vi "picoscope_910nm hitung distance_kompensasi gain.vi"() -> ()   [LabVIEW 2016]
doc: "This example demonstrates how to continuously re-generate analog output data from a buffer in your computer's memory.\n\nRefer to your device documentation for pinouts and hardware capabilities."
uses:
  <vilib>/Analysis/coordinate.llb/Angle Units.ctl
  <vilib>/Analysis/coordinate.llb/Angle Range (Degree).ctl
  <vilib>/Analysis/baseanly.llb/Mean (DBL).vi
  <vilib>/Analysis/coordinate.llb/Wrap Angle (scalar).vi
  <vilib>/measure/mascope.llb/Pulse Measurements 1 chan.vi
  <vilib>/measure/matone.llb/Extract Single Tone Information 1 Chan.vi
  <vilib>/measure/NI_MAPro.lvlib
  <vilib>/Analysis/NI_AAL_Angle.lvlib
  <vilib>/Analysis/NI_AALBase.lvlib
panel:
  in  "Channel C":T1={"Enabled"=TRUE, "DC Coupled"=FALSE, "Range"=6} {"Range" items=["10 mV", "20 mV", "50 mV", "100 mV", "200 mV", "500 mV", "1 V", "2 V", "5 V", "10 V", "20 V", "50 V ", "100 V"]}
  in  "Reset saving":bool caption="Reset"
  in  "Acquisition Settings":T2={"preTriggerSamples"=0, "postTriggerSamples"=1000, "timebase"=2, "Aggregate Data"=FALSE, "Down Sample Ratio"=1, "Four Channel Device"=TRUE, "Oversample"=1} {"Down Sample Ratio" min=1 step=1}
  in  "Channel A":T1={"Enabled"=TRUE, "DC Coupled"=FALSE, "Range"=6} {"Range" items=["10 mV", "20 mV", "50 mV", "100 mV", "200 mV", "500 mV", "1 V", "2 V", "5 V", "10 V", "20 V", "50 V ", "100 V"]}
  in  "Phase Measurement":enum32{"Square", "Sinusoidal"}(tab)
  out "Time Shift 3":dbl
  out "Pulse center 3":dbl
  out "Pulse Center 2":dbl
  out "Phase Shift 2":dbl
  out "Ref frequency":dbl format="%.2p"
  out "Signal frequency":dbl format="%.2p"
  out "Amp A":dbl format="%.2g"
  out "Amp C":dbl format="%_3g"
  out "Phase total":dbl format="%#_4g"
  out "Phase 2 M":dbl format="%0.2f"
  out "Phase 10 M":dbl format="%0.2f"
  out "Validation":string="not range"
  out "Distance (m)":dbl format="%#.3g"
  in  "Enable Av_Gain":bool
  in  "Save":bool caption="Enable"
  out "Waveform Graph":dbl[][](graph) caption="Output Waveform"
  in  "Stop":bool
  out "phase sbl":dbl
  out "Phase Shift (deg)":dbl
  out "phase 2 (2M)":dbl
  out "phase 1 (10M)":dbl
  out "mean phase 10 M":dbl format="%0.2f"
  out "Array 2":dbl[](array[numeric])
  out "number 2":u32
  out "mean phase 2 M":dbl format="%0.2f"
  out "Array":dbl[](array[numeric])
  out "Phase signal":dbl
  out "number":u32
  out "appended array":bool[](array[boolean])
  out "DC RMS":dbl format="%#_3g"
  out "Data out":dbl[](array[numeric])
  out "Phase Signal ref":dbl
  in  "Channel D Settings":T1={"Enabled"=FALSE, "DC Coupled"=TRUE, "Range"=6} {"Range" items=["10 mV", "20 mV", "50 mV", "100 mV", "200 mV", "500 mV", "1 V", "2 V", "5 V", "10 V", "20 V", "50 V ", "100 V"]}
  in  "Channel B Settings":T1={"Enabled"=FALSE, "DC Coupled"=FALSE, "Range"=6} {"Range" items=["10 mV", "20 mV", "50 mV", "100 mV", "200 mV", "500 mV", "1 V", "2 V", "5 V", "10 V", "20 V", "50 V ", "100 V"]}
  # "median"
  # "Channel Settings"
  # "Trigger Settings"
  # "1   2   4   8   16  32 64 128  256 512 1024  2028"
  # "OPI i-ToF LiDAR\nResearch Center for Photonics - BRIN"
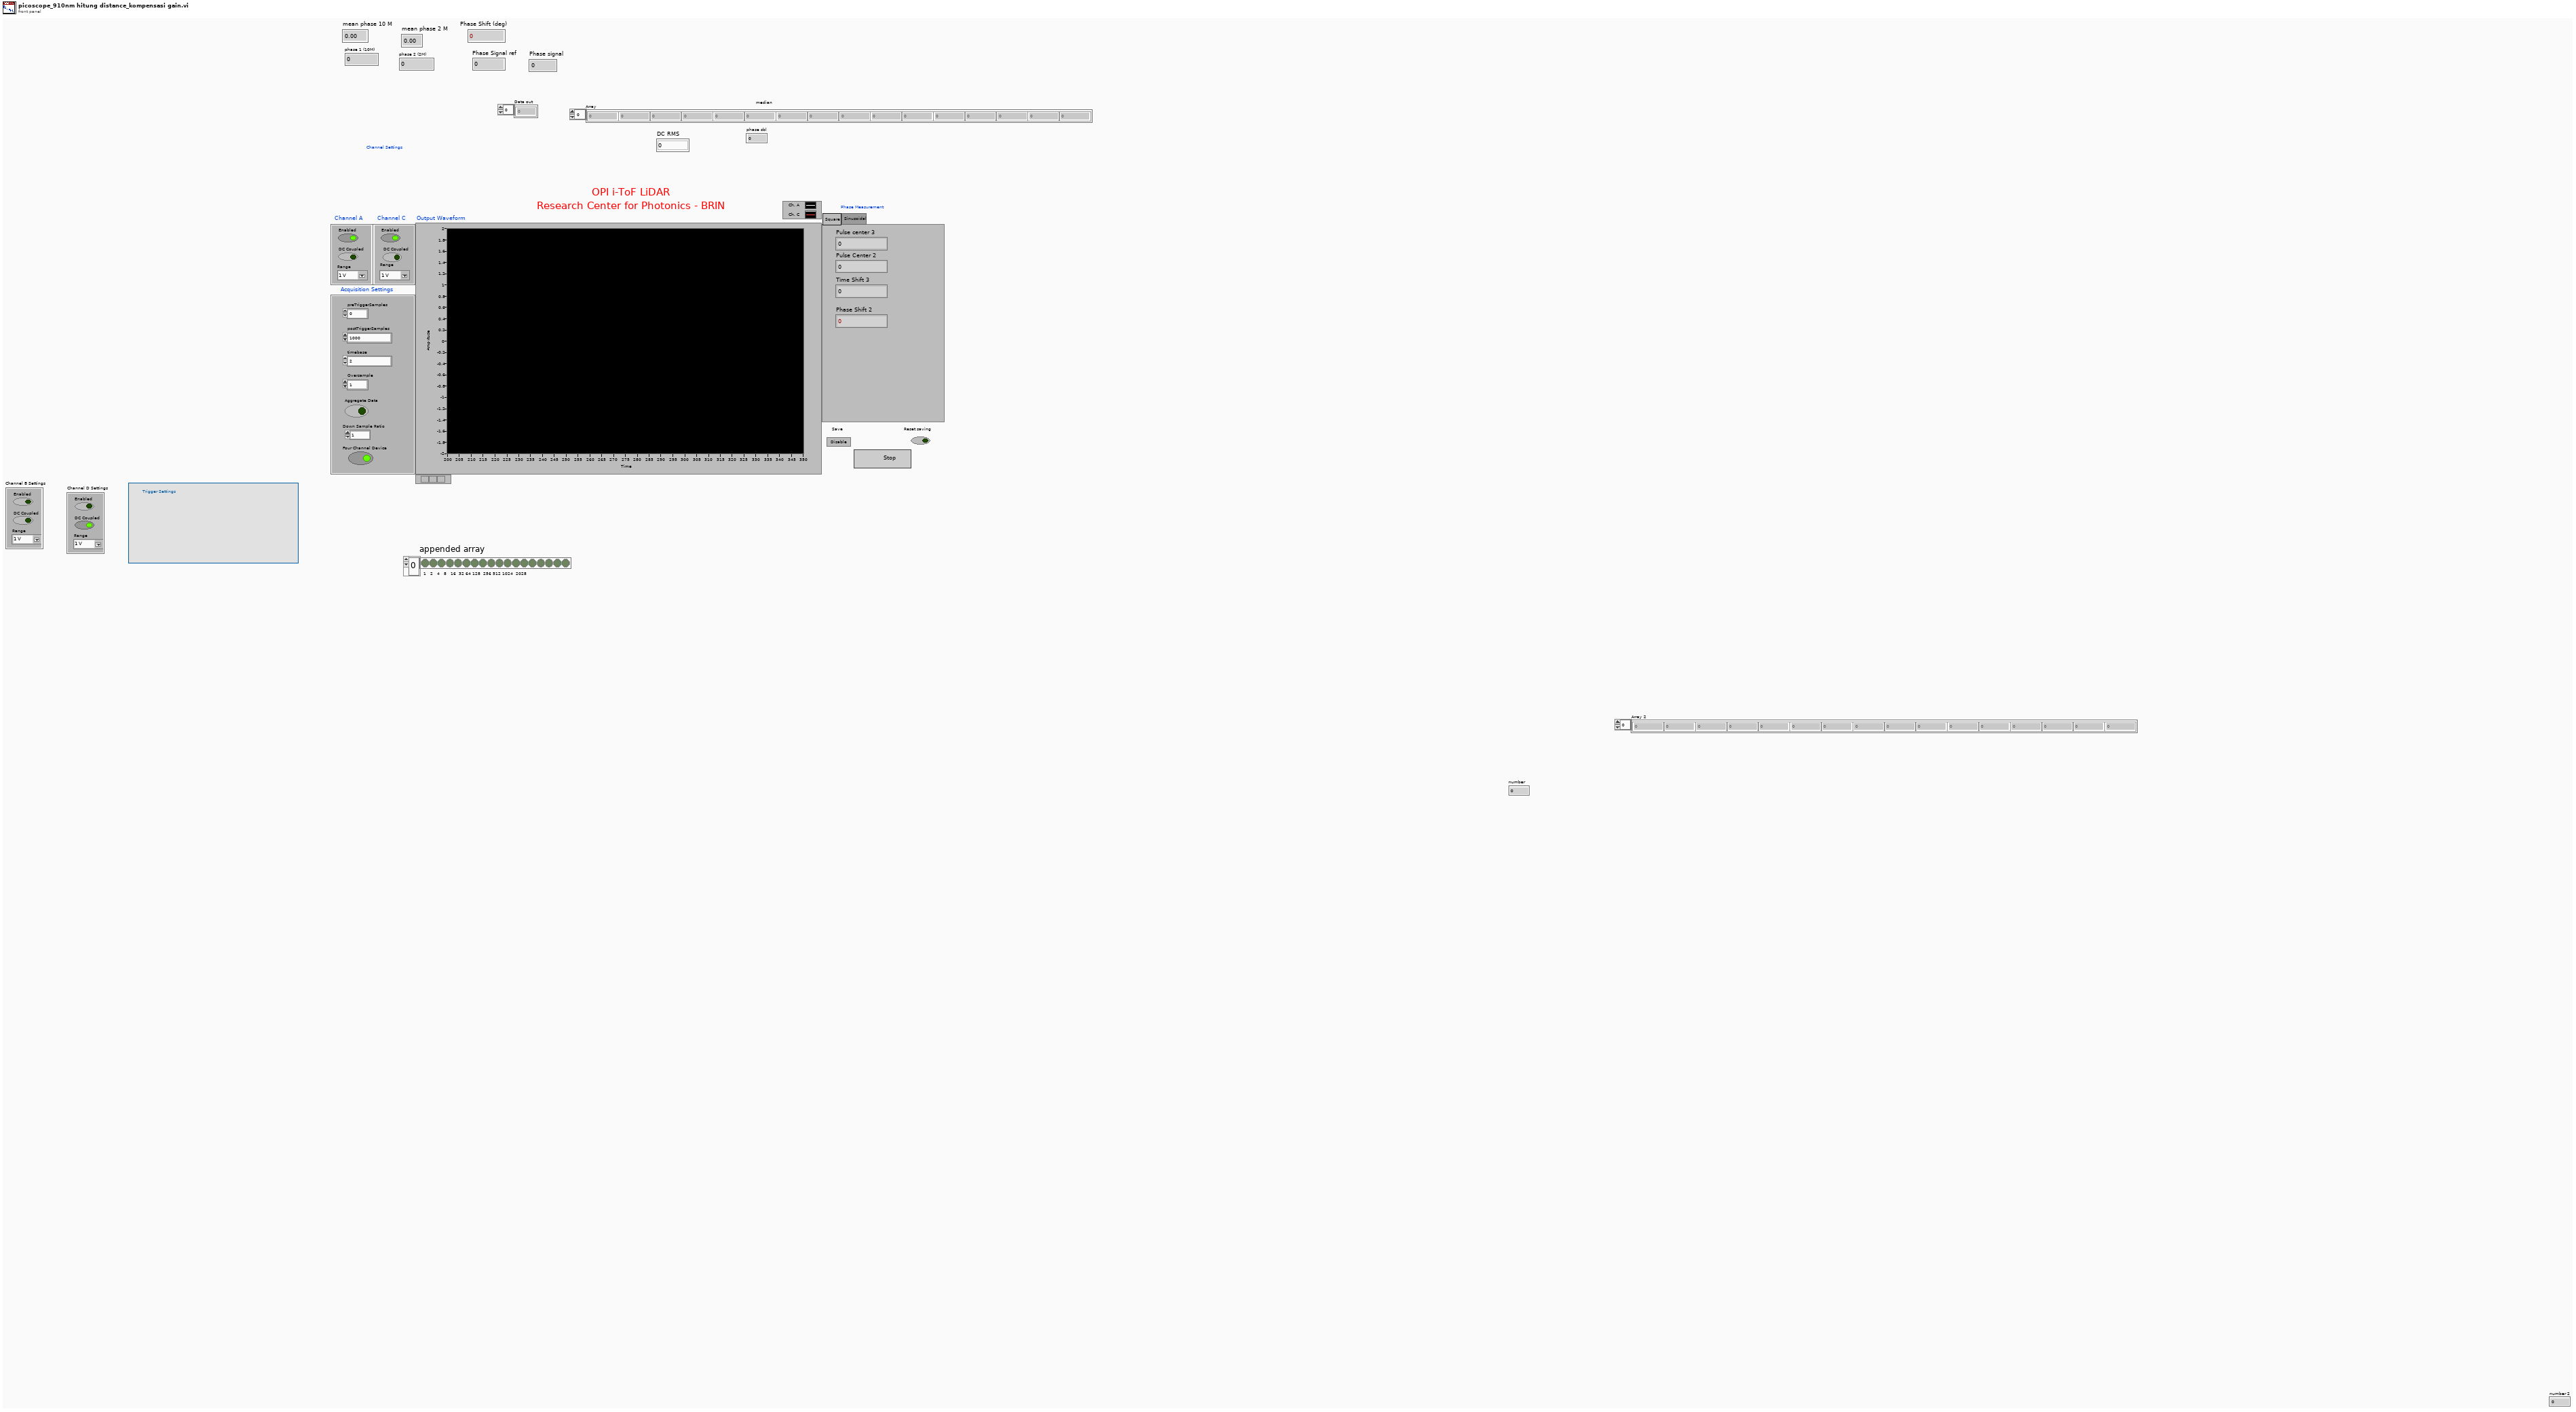
[diagram p1: front panel]
types:
  T1 = cluster{"Enabled":bool, "DC Coupled":bool, "Range":u16}
  T2 = cluster{"preTriggerSamples":i32, "postTriggerSamples":i32, "timebase":u32, "Aggregate Data":bool, "Down Sample Ratio":u32, "Four Channel Device":bool, "Oversample":i16}
  T3 = cluster{"Channel D Buffer":i16[], "Channel C Buffer":i16[], "Channel B Buffer":i16[], "Channel A Buffer":i16[]}
  T4 = cluster{"pulse center":dbl, "ref levels":cluster{"high ref level":dbl, "mid ref level":dbl, "low ref level":dbl, "ref units":u16}}
  T5 = typedef "NI_AAL_Angle.lvlib/Angle Range (Degree).ctl" = u16
  T6 = typedef "NI_AAL_Angle.lvlib/Angle Units.ctl" = i32
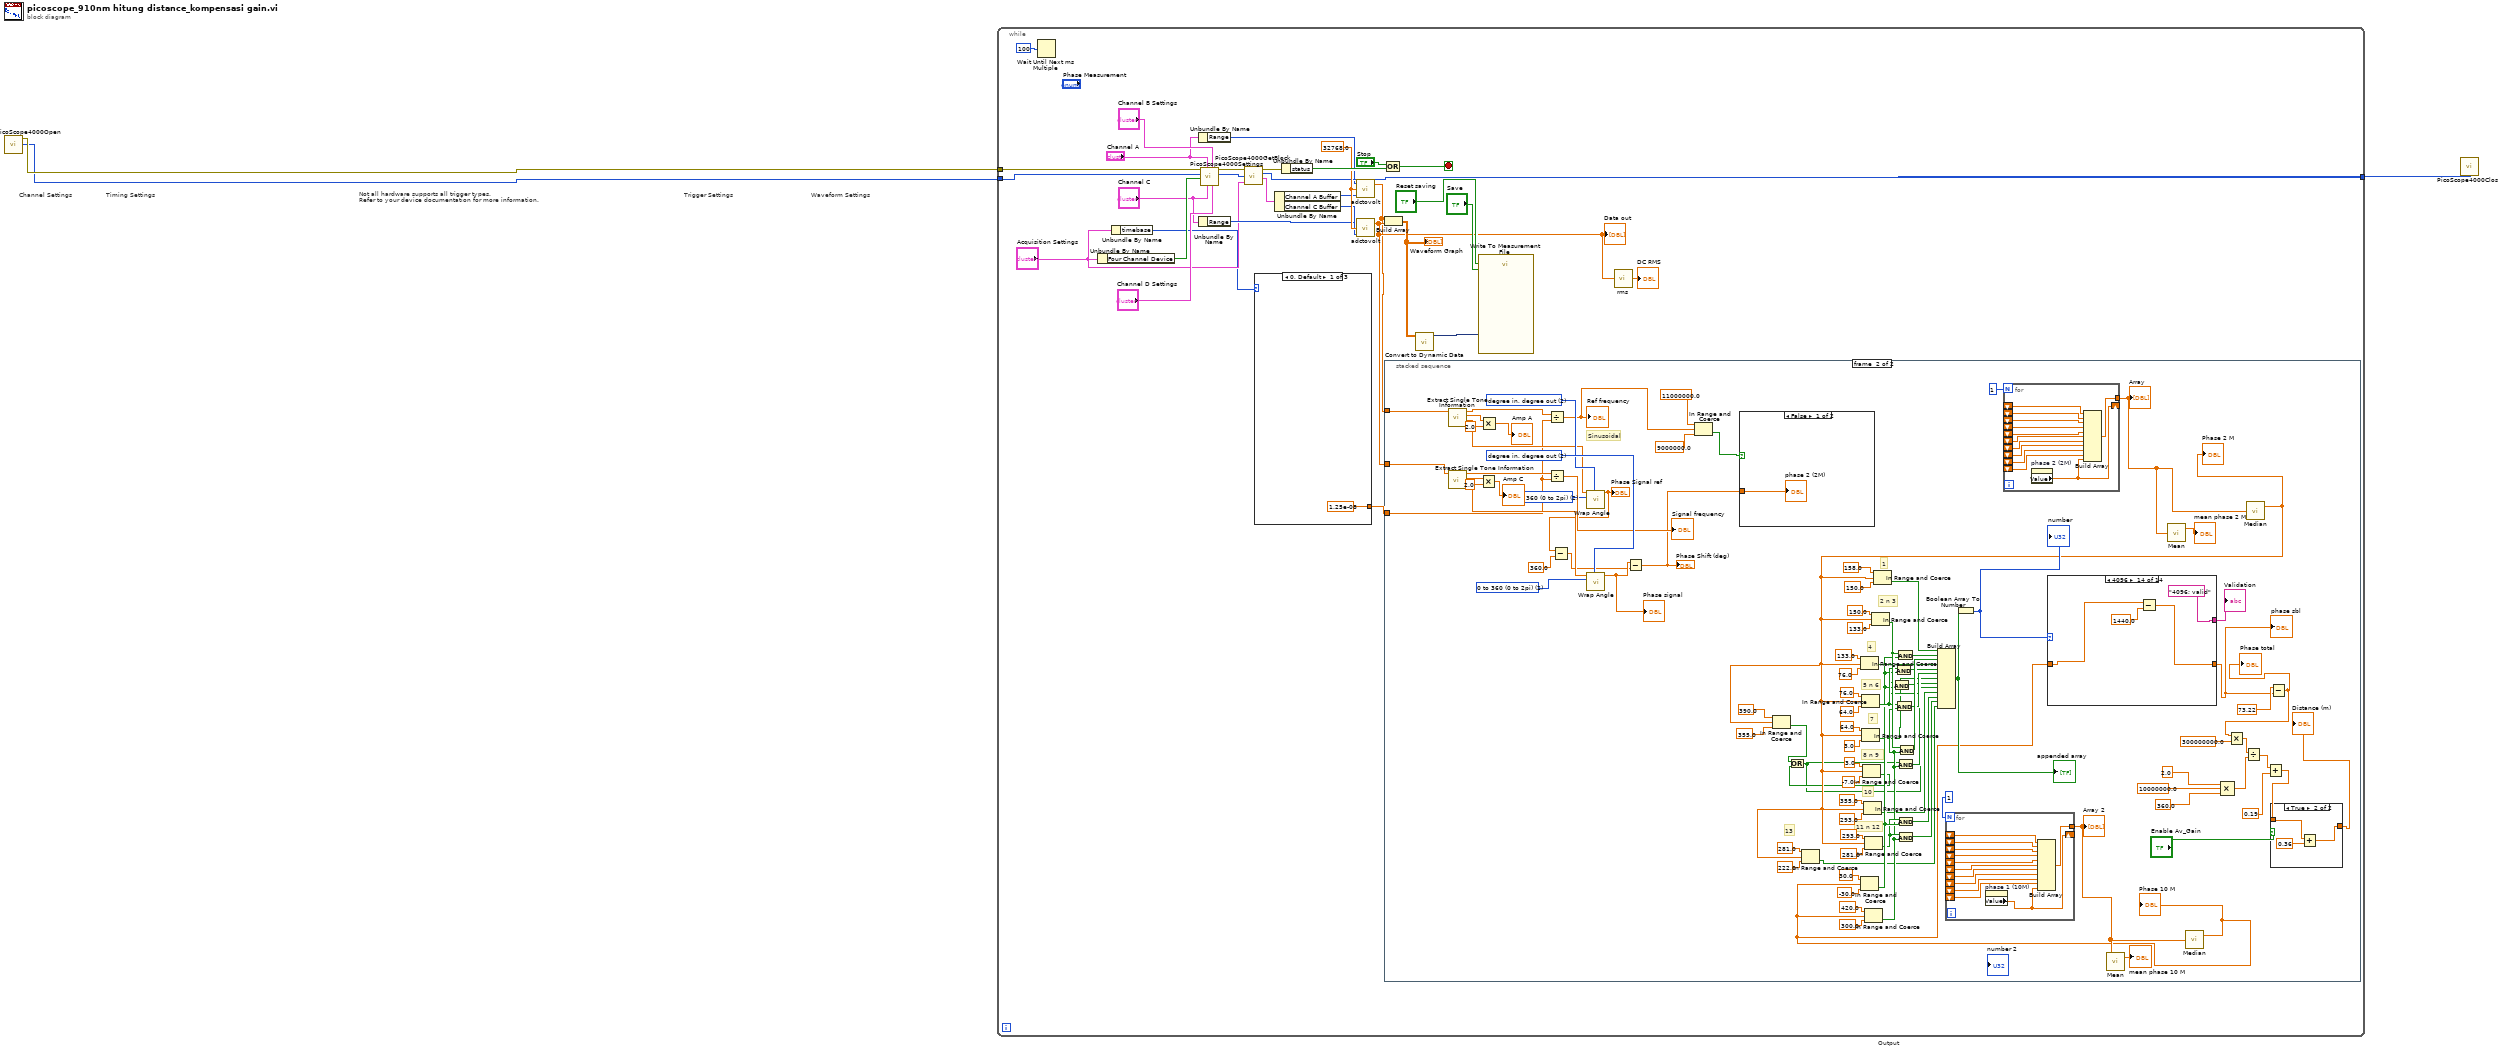
[diagram p0: block diagram]
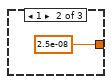
[diagram p2: hidden frame]
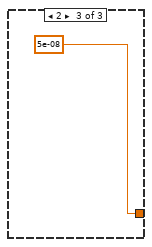
[diagram p3: hidden frame]
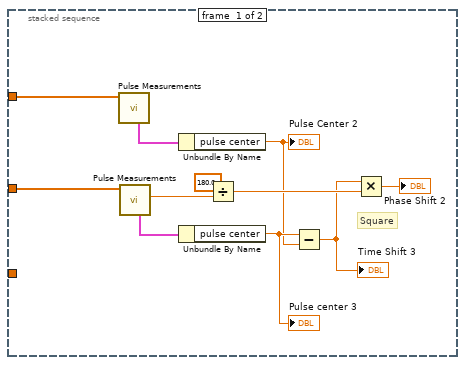
[diagram p4: hidden frame]
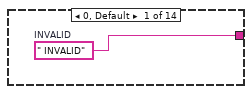
[diagram p6: hidden frame]
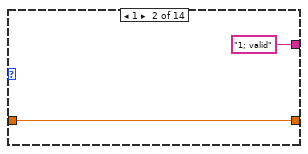
[diagram p7: hidden frame]
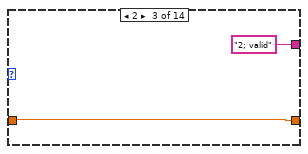
[diagram p8: hidden frame]
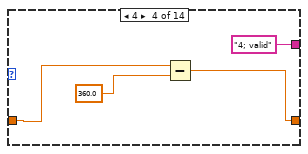
[diagram p9: hidden frame]
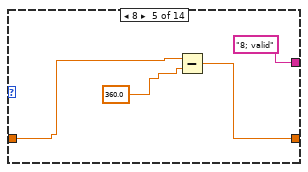
[diagram p10: hidden frame]
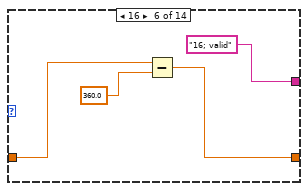
[diagram p11: hidden frame]
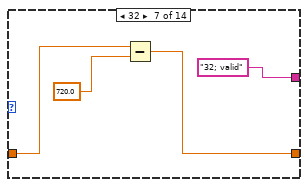
[diagram p12: hidden frame]
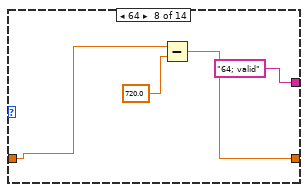
[diagram p13: hidden frame]
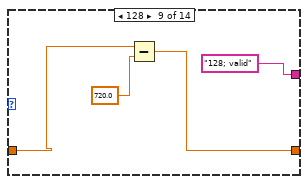
[diagram p14: hidden frame]
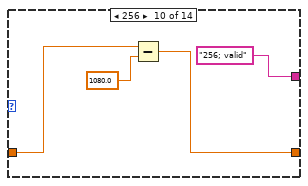
[diagram p15: hidden frame]
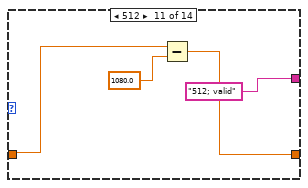
[diagram p16: hidden frame]
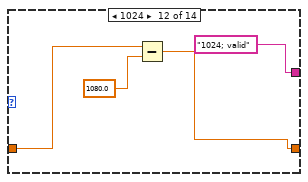
[diagram p17: hidden frame]
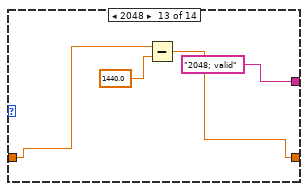
[diagram p18: hidden frame]
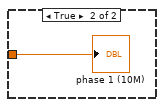
[diagram p19: hidden frame]
diagram:
  # "Not all hardware supports all trigger types.\nRefer to your device documentation for more information."
  # "Trigger Settings"
  # "Output"
  # "Waveform Settings"
  # "Timing Settings"
  # "Channel Settings"
  n1 = call "PicoScope4000Open.vi"() -> ("error out"=w2:errorcluster, "handle"=w1:i16)  [unwired: 1 in, 1 out]
  n2 = while {
    tunnel: w2 -> [w17]
    tunnel: w1 -> [w15]
    tunnel: [w24] -> w3
    stop <- w31 stop-if-true
    w27 = 32768.0 ("Max_adc")
    n3 = Wait Until Next ms Multiple(millisecond multiple=u32 100) -> ()  [unwired: 1 out]
    n4 = Unbundle By Name("Acquisition Settings") -> ("Four Channel Device"=w13:bool)
    n5 = Unbundle By Name("Acquisition Settings") -> ("timebase"=w8:u32)
    n6 = Unbundle By Name("Channel A") -> ("Range"=w18:u16)
    n7 = Unbundle By Name("Channel C") -> ("Range"=w10:u16)
    n8 = call "PicoScope4000Settings.vi"("Channel D Settings"="Channel D Settings", "Channel B Settings"="Channel B Settings", "Channel C Settings"="Channel C", "Channel A Settings"="Channel A", "Four Channel Device?"=w13, "handle in"=w15, "error in"=w17) -> ("handle out"=w14:i16, "error out"=w16:errorcluster)  [unwired: 3 in]
    n9 = call "PicoScope4000GetBlock.vi"("error in"=w16, "handle in"=w14, "Acquisition Settings"="Acquisition Settings") -> ("error out"=w23:errorcluster, "handle out"=w24:i16, "Buffers (Max or non-aggregated)"=w28:T3)  [unwired: 3 in, 2 out]
    n10 = case shown="0, Default" w8 {
      tunnel: [1.25e-08 2.5e-08 5e-08] -> w7
      frame 0, Default {
      }
      frame 1 {
      }
      frame 2 {
      }
    }
    n11 = Unbundle By Name(w28) -> ("Channel A Buffer"=w26:i16[], "Channel C Buffer"=w25:i16[])
    n12 = Unbundle By Name(w23) -> ("status"=w32:bool)
    n13 = call "adctovolt.vi"("Data in"=w26, "Max_adc"=w27, "Range Index"=w18) -> ("Data out"=w4:dbl[])  [unwired: 1 in]
    n14 = call "adctovolt.vi"("Data in"=w25, "Max_adc"=w27, "Range Index"=w10) -> ("Data out"=w6:dbl[])  [unwired: 1 in]
    "Data out" <- w6
    n15 = Build Array(w4, w6) -> (w22:dbl[][])
    "Waveform Graph" <- w22
    n16 = stacked-sequence {
      tunnel: w4 -> [w43 w145]
      tunnel: w6 -> [w42 w144]
      tunnel: w7 -> [_ w136]
      frame #0 {
        # "Square"
        n17 = call-poly <vilib>:"Pulse Measurements.vi"("signal in"=w43) -> ("measurement info"=w46:T4)  [unwired: 3 in, 7 out]
        n18 = call-poly <vilib>:"Pulse Measurements.vi"("signal in"=w42) -> ("pulse duration"=w44:dbl, "measurement info"=w45:T4)  [unwired: 3 in, 6 out]
        n19 = Unbundle By Name(w46) -> ("pulse center"=w38:dbl)
        "Pulse Center 2" <- w38
        n20 = Unbundle By Name(w45) -> ("pulse center"=w39:dbl)
        "Pulse center 3" <- w39
        n21 = Divide(x=180.0 ("y"), y=w44) -> (x/y=w48:dbl)
        n22 = Subtract(x=w39, y=w38) -> (x-y=w41:dbl)
        "Time Shift 3" <- w41
        n23 = Multiply(x=w41, y=w48) -> (x*y=→"Phase Shift 2":dbl)
      }
      frame #1 {
        w108 = T5 2 items=["none", "-180 to 180 (-pi to pi)", "0 to 360 (0 to 2pi)"] ("angle range")
        w109 = T5 2 items=["none", "-180 to 180 (-pi to pi)", "0 to 360 (0 to 2pi)"] ("angle range")
        w141 = T6 2 items=["radian in, radian out", "radian in, degree out", "degree in, degree out", "degree in, radian out"] ("angle units")
        w143 = T6 2 items=["radian in, radian out", "radian in, degree out", "degree in, degree out", "degree in, radian out"] ("angle units")
        # "13"
        # "11 n 12"
        # "10"
        # "8 n 9"
        # "7"
        # "5 n 6"
        # "4"
        # "2 n 3"
        # "1"
        # "Sinusoidal"
        n24 = call-poly <vilib>:"Extract Single Tone Information.vi"("time signal in"=w145) -> ("detected phase (deg)"=w140:dbl, "detected amplitude"=w135:dbl, "detected frequency"=w137:dbl)  [unwired: 3 in, 5 out]
        n25 = call-poly <vilib>:"Extract Single Tone Information.vi"("time signal in"=w144) -> ("detected phase (deg)"=w142:dbl, "detected amplitude"=w132:dbl, "detected frequency"=w139:dbl)  [unwired: 3 in, 5 out]
        n26 = Multiply(x=w132, y=2.0) -> (x*y=→"Amp C":dbl)
        n27 = Multiply(x=w135, y=2.0) -> (x*y=→"Amp A":dbl)
        n28 = Divide(x=w137, y=w136) -> (x/y=w128:dbl)
        "Ref frequency" <- w128
        n29 = Divide(x=w139, y=w136) -> (x/y=→"Signal frequency":dbl)
        n30 = call-poly <vilib>:"Wrap Angle.vi"("angle units"=w141, "angle range"=w108, "angle in"=w140) -> ("angle out"=w72:dbl)  [unwired: 7 in, 1 out]
        "Phase Signal ref" <- w72
        n31 = Subtract(x=w72, y=360.0) -> (x-y=w71:dbl)
        n32 = call-poly <vilib>:"Wrap Angle.vi"("angle units"=w143, "angle range"=w109, "angle in"=w142) -> ("angle out"=w74:dbl)  [unwired: 7 in, 1 out]
        "Phase signal" <- w74
        n33 = Subtract(x=w74, y=w71) -> (x-y=w70:dbl)
        "Phase Shift (deg)" <- w70
        n34 = In Range and Coerce(upper limit=11000000.0, x=w128, lower limit=9000000.0) -> (In Range?=w129:bool)  [unwired: 1 out]
        n35 = case shown="False" w129 {
          tunnel: w70 -> [w223 w224]
          frame False {
            "phase 2 (2M)" <- w223
          }
          frame True {
            "phase 1 (10M)" <- w224
          }
        }
        n36 = for {
          N: 1 -> [_]
          shift-right: [w150] -> _
          shift-left: _ -> [w158]
          tunnel: [w161] -> w103
          shift-left: _ -> [w157]
          shift-left: _ -> [w156]
          shift-left: _ -> [w159]
          shift-left: _ -> [w160]
          shift-left: _ -> [w155]
          shift-left: _ -> [w154]
          shift-left: _ -> [w153]
          shift-left: _ -> [w152]
          shift-left: _ -> [w151]
          n37 = property on="phase 1 (10M)" class="DigNum (strict)"() -> ("Value"=w150:dbl)  [unwired: 2 in, 2 out]
          n38 = Build Array(w160, w159, w158, w157, w156, w155, w154, w153, w152, w151, w150) -> (w161:dbl[])
        }
        "Array 2" <- w103
        n39 = for {
          N: 1 -> [_]
          shift-right: [w172] -> _
          shift-left: _ -> [w169]
          tunnel: [w173] -> w106
          shift-left: _ -> [w168]
          shift-left: _ -> [w167]
          shift-left: _ -> [w170]
          shift-left: _ -> [w171]
          shift-left: _ -> [w166]
          shift-left: _ -> [w165]
          shift-left: _ -> [w164]
          shift-left: _ -> [w163]
          shift-left: _ -> [w162]
          n40 = property on="phase 2 (2M)" class="DigNum (strict)"() -> ("Value"=w172:dbl)  [unwired: 2 in, 2 out]
          n41 = Build Array(w171, w170, w169, w168, w167, w166, w165, w164, w163, w162, w172) -> (w173:dbl[])
        }
        "Array" <- w106
        n42 = call-poly <vilib>:"Mean.vi"("X"=w103) -> ("mean"=→"mean phase 10 M":dbl)  [unwired: 1 out]
        n43 = call-poly <vilib>:"Mean.vi"("X"=w106) -> ("mean"=→"mean phase 2 M":dbl)  [unwired: 1 out]
        n44 = call <vilib>:"Median.vi"("X"=w103) -> ("median"=w69:dbl)  [unwired: 1 out]
        "Phase 10 M" <- w69
        n45 = In Range and Coerce(upper limit=30.0, x=w69, lower limit=-30.0) -> (In Range?=w83:bool)  [unwired: 1 out]
        n46 = In Range and Coerce(upper limit=420.0, x=w69, lower limit=300.0) -> (In Range?=w80:bool)  [unwired: 1 out]
        n47 = Compound Arithmetic op=MULTIPLY(2.0 ("value"), 10000000.0 ("value"), 360.0 ("value")) -> (w110:dbl)
        n48 = call <vilib>:"Median.vi"("X"=w106) -> ("median"=w63:dbl)  [unwired: 1 out]
        "Phase 2 M" <- w63
        n49 = In Range and Coerce(upper limit=390.0, x=w63, lower limit=355.0) -> (In Range?=w60:bool)  [unwired: 1 out]
        n50 = In Range and Coerce(upper limit=281.0, x=w63, lower limit=222.0) -> (In Range?=w76:bool)  [unwired: 1 out]
        n51 = In Range and Coerce(upper limit=133.0, x=w63, lower limit=76.0) -> (In Range?=w99:bool)  [unwired: 1 out]
        n52 = In Range and Coerce(upper limit=76.0, x=w63, lower limit=64.0) -> (In Range?=w94:bool)  [unwired: 1 out]
        n53 = In Range and Coerce(upper limit=64.0, x=w63, lower limit=3.0) -> (In Range?=w53:bool)  [unwired: 1 out]
        n54 = In Range and Coerce(upper limit=3.0, x=w63, lower limit=-7.0) -> (In Range?=w62:bool)  [unwired: 1 out]
        n55 = Or(x=w60, y=w62) -> (x .or. y?=w61:bool)
        n56 = In Range and Coerce(upper limit=355.0, x=w63, lower limit=293.0) -> (In Range?=w52:bool)  [unwired: 1 out]
        n57 = In Range and Coerce(upper limit=293.0, x=w63, lower limit=281.0) -> (In Range?=w81:bool)  [unwired: 1 out]
        n58 = In Range and Coerce(upper limit=150.0, x=w63, lower limit=133.0) -> (In Range?=w116:bool)  [unwired: 1 out]
        n59 = In Range and Coerce(upper limit=158.0 ("y"), x=w63, lower limit=150.0 ("y")) -> (In Range?=w66:bool)  [unwired: 1 out]
        n60 = And(x=w61, y=w83) -> (x .and. y?=w89:bool)
        n61 = And(x=w94, y=w83) -> (x .and. y?=w96:bool)
        n62 = And(x=w94, y=w80) -> (x .and. y?=w95:bool)
        n63 = And(x=w116, y=w83) -> (x .and. y?=w117:bool)
        n64 = And(x=w61, y=w80) -> (x .and. y?=w88:bool)
        n65 = And(x=w81, y=w83) -> (x .and. y?=w82:bool)
        n66 = And(x=w81, y=w80) -> (x .and. y?=w79:bool)
        n67 = And(x=w116, y=w80) -> (x .and. y?=w115:bool)
        n68 = Build Array(w66, w117, w115, w99, w96, w95, w53, w89, w88, w52, w82, w79, w76) -> (w123:bool[])
        "appended array" <- w123
        n69 = Boolean Array To Number(Boolean array=w123) -> (number=w122:u32)
        "number" <- w122
        n70 = case shown="4096" w122 {
          tunnel: w69 -> [_ w175 w178 w180 w184 w188 w192 w195 w199 w203 w207 w211 w215 w219]
          tunnel: [_ w175 w178 w182 w186 w190 w194 w198 w202 w206 w210 w214 w218 w222] -> w58
          tunnel: [w174 "1; valid" "2; valid" "4; valid" "8; valid" "16; valid" "32; valid" "64; valid" "128; valid" "256; valid" "512; valid" "1024; valid" "2048; valid" "4096; valid"] -> w75
          frame 0, Default {
            w174 = " INVALID"  # INVALID
          }
          frame 1 {
          }
          frame 2 {
          }
          frame 4 {
            n71 = Subtract(x=w180, y=360.0 ("x")) -> (x-y=w182:dbl)
          }
          frame 8 {
            n72 = Subtract(x=w184, y=360.0 ("x")) -> (x-y=w186:dbl)
          }
          frame 16 {
            n73 = Subtract(x=w188, y=360.0 ("x")) -> (x-y=w190:dbl)
          }
          frame 32 {
            n74 = Subtract(x=w192, y=720.0 ("x")) -> (x-y=w194:dbl)
          }
          frame 64 {
            n75 = Subtract(x=w195, y=720.0 ("x")) -> (x-y=w198:dbl)
          }
          frame 128 {
            n76 = Subtract(x=w199, y=720.0 ("x")) -> (x-y=w202:dbl)
          }
          frame 256 {
            n77 = Subtract(x=w203, y=1080.0 ("x")) -> (x-y=w206:dbl)
          }
          frame 512 {
            n78 = Subtract(x=w207, y=1080.0 ("x")) -> (x-y=w210:dbl)
          }
          frame 1024 {
            n79 = Subtract(x=w211, y=1080.0 ("x")) -> (x-y=w214:dbl)
          }
          frame 2048 {
            n80 = Subtract(x=w215, y=1440.0 ("x")) -> (x-y=w218:dbl)
          }
          frame 4096 {
            n81 = Subtract(x=w219, y=1440.0 ("x")) -> (x-y=w222:dbl)
          }
        }
        "Validation" <- w75
        "phase sbl" <- w58
        n82 = Subtract(x=73.22 ("y"), y=w58) -> (x-y=w57:dbl)
        "Phase total" <- w57
        n83 = Multiply(x=w57, y=300000000.0) -> (x*y=w111:dbl)
        n84 = Divide(x=w111, y=w110) -> (x/y=w56:dbl)
        n85 = Add(x=w56, y=0.19) -> (x+y=w50:dbl)
        n86 = case shown="True" "Enable Av_Gain" {
          tunnel: [w146 w147] -> w49
          tunnel: w50 -> [w146 w149]
          frame False {
          }
          frame True {
            n87 = Add(x=w149, y=0.36) -> (x+y=w147:dbl)
          }
        }
        "Distance (m)" <- w49
      }
    }
    n88 = Compound Arithmetic op=OR("Stop", w32) -> (w31:bool)
    n89 = call "Convert to Dynamic Data"("2D Array"=w22) -> ("Dynamic Data Type"=w29:dynamicdata)  [unwired: 3 in]
    n90 = call "Write To Measurement File"("Signals"=w29, "Reset"="Reset saving", "Enable"="Save") -> ()  [unwired: 14 in, 3 out]
    n91 = call <userlib>:"rms.vi"("Float array"=w6) -> ("RMS value"=→"DC RMS":dbl)  [unwired: 4 in]
  }
  n92 = call "PicoScope4000Close.vi"("handle"=w3) -> ()
